vi "Ximea get frame and display.vi"(8 "error in (no error)":errorcluster, 10 "Image In":T1, 11 "xiCam In":refnum<k24>) -> (0 "error out":errorcluster, 1 "FrameNumber":u32, 2 "Image Out":T1, 3 "xiCam Out":refnum<k24>)   [LabVIEW 2016]
uses:
  C:/Users/Ries Lab/Documents/Microscope Control from Sheng Account/Microscope-Control/Device Library/Cameras/Ximea/xiLIB_64bit/xiLIB/xiCamLib/API/x64/xiApi.NETX64.dll
  xiLIB_64bit/xiLIB/xiCamLib/API/x64/xiApi.NETX64.dll
  <vilib>/vision/Image Controls.llb/IMAQ Image.ctl
  Camera Controls/Camera IMAQ Key Info.ctl
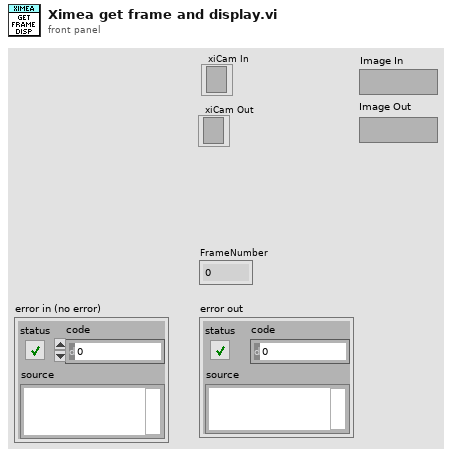
[diagram p1: front panel]
types:
  T1 = typedef "IMAQ Image.ctl" = refnum<image>
  T2 = typedef "Camera IMAQ Key Info.ctl" = cluster{"Frame":u32, "Sensor Height":i32, "Sensor Width":i32, "ROI Height":i32, "ROI Width":i32, "ROI Enable?":bool, "Bit per Pixel":u8}
  T3 = typedef "xiImageMng - Attributes.ctl" = cluster{"WIDTH":i32, "HEIGHT":i32, "IMG_FORMAT":T4}
  T4 = typedef "IMG_DATA_FORMAT.ctl" = enum16{"MONO8", "MONO16", "RGB24", "RGB32", "RGBPLANAR", "RAW8", "RAW16"}
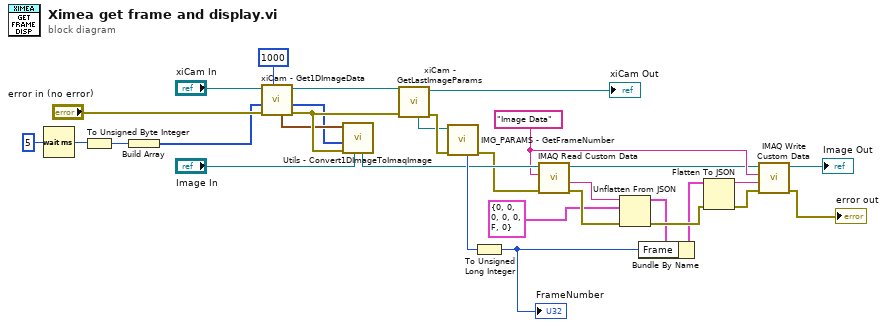
[diagram p0: block diagram]
diagram:
  w19 = "Image Data" ("Key")
  n1 = Wait (ms)(milliseconds to wait=u32 5) -> (millisecond timer value=w3:u32)
  n2 = To Unsigned Byte Integer(number=w3) -> (unsigned 8bit integer=w2:u8)
  n3 = Build Array(w2) -> (w1:u8[])
  n4 = call "xiCam - Get1DImageData.vi"("timeout"=1000, "error in (no error)"="error in (no error)", "1DImageData In"=w1, "xiCam In"="xiCam In") -> ("error out"=w25:errorcluster, "1DImageData Out"=w9:u8[], "xiCam Out"=w11:refnum<k24>, "Image Properites"=w10:T3)  [unwired: 4 in]
  n5 = call "Utils - Convert1DImageToImaqImage.vi"("Image In"="Image In", "error in (no error)"=w25, "1DImageData In"=w9, "Image Properties In"=w10) -> ("Image Out"=w30:T1)  [unwired: 5 in, 2 out]
  n6 = call "xiCam - GetLastImageParams.vi"("error in (no error)"=w25, "xiCam In"=w11) -> ("error out"=w26:errorcluster, "xiCam Out"=→"xiCam Out":refnum<k24>, "GetLastImageParams"=w12:refnum<k24>)  [unwired: 7 in]
  n7 = call "IMG_PARAMS - GetFrameNumber.vi"("error in (no error)"=w26, "xiApi.NET.ImgParams"=w12) -> ("error out"=w27:errorcluster, "FrameNumber"=w31:i32)  [unwired: 7 in, 1 out]
  n8 = To Unsigned Long Integer(number=w31) -> (unsigned 32bit integer=w6:u32)
  "FrameNumber" <- w6
  n9 = call "IMAQ Read Custom Data"("error in (no error)"=w27, "Key"=w19, "Image"=w30) -> ("error out"=w20:errorcluster, "Custom Data Out"=w15:string, "Image (duplicate)"=w13:T1)  [unwired: 6 in]
  n10 = Unflatten From JSON(JSON string=w15, type and defaults=T2 {"Frame"=0, "Sensor Height"=0, "Sensor Width"=0, "ROI Height"=0, "ROI Width"=0, "ROI Enable?"=FALSE, "Bit per Pixel"=0} ("Camera IMAQ Key Info"), error in (no error)=w20) -> (value=w16:T2, error out=w21:errorcluster)  [unwired: 4 in]
  n11 = Bundle By Name(cluster=w16, "Frame"=w6) -> (w17:T2)
  n12 = Flatten To JSON(anything=w17, error in (no error)=w21) -> (JSON string=w18:string, 11:w22:errorcluster)  [unwired: 1 in]
  n13 = call "IMAQ Write Custom Data"("error in (no error)"=w22, "Custom Data In"=w18, "Key"=w19, "Image"=w13) -> ("error out"=→"error out":errorcluster, "Image Out"=→"Image Out":T1)  [unwired: 6 in]
